vi "Get Port Direction.vi"(8 "error in":errorcluster, 11 "port ref in":T2 format="%.0x") -> (0 "error out":errorcluster, 2 "direction":T1, 3 "port ref out":T2 format="%.0x")   [LabVIEW 2020, in "ARINC 429 Scripting.lvlib"]
uses:
  ARINC 429 Scripting.lvlib
  <vilib>/NI VeriStand/Custom Device API/Custom Device Item Ref.ctl
  Shared/Direction.ctl
  Ballard/Constants.vi
  Ballard/Ballard ARINC 429 Scripting.lvlib
  <vilib>/NI VeriStand/Custom Device API/Custom Device API.lvlib
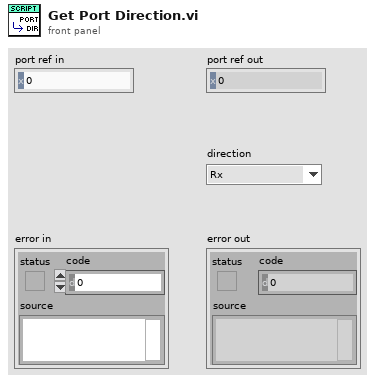
[diagram p1: front panel]
types:
  T1 = typedef "Direction.ctl" = enum16{"Rx", "Tx"}
  T2 = typedef "Custom Device API.lvlib/Custom Device Item Ref.ctl" = u64
  T3 = typedef "Custom Device API.lvlib/Custom Device Item Info.ctl" = cluster{"Name":string, "Is Channel":bool, "GUID":string, "Is Waveform":bool}
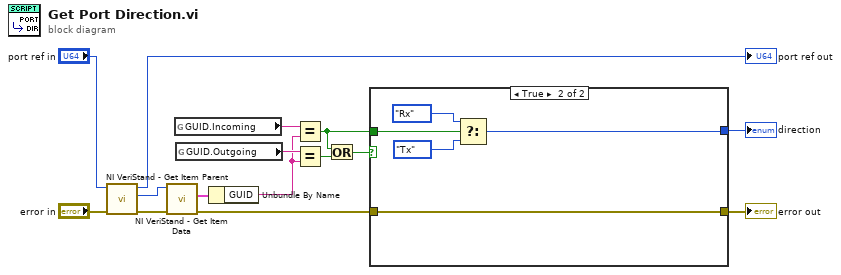
[diagram p0: block diagram]
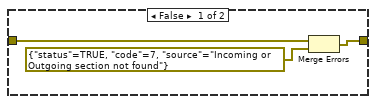
[diagram p2: hidden frame]
diagram:
  n1 = call <vilib>:"NI VeriStand - Get Item Parent.vi"("error in (no error)"="error in", "Item Ref in"="port ref in") -> ("error out"=w13:errorcluster, "Parent Ref"=w11:T2, "Item Ref out"=→"port ref out":T2)  [unwired: 6 in, 1 out]
  n2 = call <vilib>:"NI VeriStand - Get Item Data.vi"("error in (no error)"=w13, "Item Ref in"=w11) -> ("error out"=w4:errorcluster, "Item Info"=w10:T3)  [unwired: 6 in, 2 out]
  n3 = global read "Constants.vi" "GUID.Incoming"() -> (w8:string)
  n4 = global read "Constants.vi" "GUID.Outgoing"() -> (w9:string)
  n5 = Unbundle By Name(w10) -> ("GUID"=w7:string)
  n6 = Equal?(x=w8, y=w7) -> (x = y?=w2:bool)
  n7 = Equal?(x=w9, y=w7) -> (x = y?=w6:bool)
  n8 = Or(x=w2, y=w6) -> (x .or. y?=w5:bool)
  n9 = case shown="True" w5 {
    tunnel: w4 -> [w18 w23]
    tunnel: [w17 w23] -> w3
    tunnel: w2 -> [_ w22]
    tunnel: [_ w19] -> w1
    frame False {
      n10 = Merge Errors(w18, errorcluster {"status"=TRUE, "code"=7, "source"="Incoming or Outgoing section not found"} ("error in")) -> (w17:errorcluster)
    }
    frame True {
      n11 = Select(t=Direction."Rx" ("direction"), s=w22, f=Direction."Tx" ("direction")) -> (s? t:f=w19:T1)
    }
  }
  "error out" <- w3
  "direction" <- w1
